vi "autosize_columns_for_text.vi"(7 "font":T1, 11 "array_to_autosize":string[][](array[string])) -> (3 "column_widths":i16[](array[numeric]))   [LabVIEW 2019]
doc: "This VI resizes each column of the table specified by Table Ref based on the widest entry of the column. Additionally, if Resize Table? is TRUE, the VI will set the table width based on the number of populated columns."
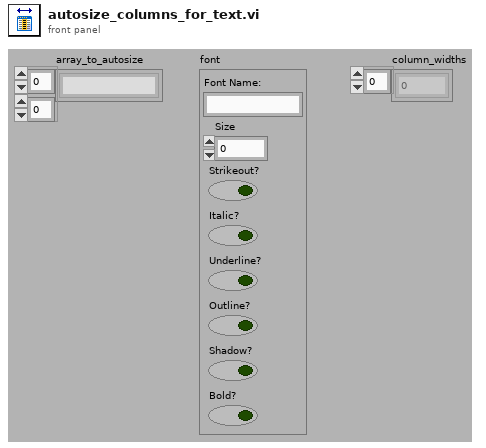
[diagram p1: front panel]
types:
  T1 = cluster{"Font Name:":string, "Size":i16, "Strikeout?":bool, "Italic?":bool, "Underline?":bool, "Outline?":bool, "Shadow?":bool, "Bold?":bool}
  T2 = enum16{"User-specified Font", "Application Font", "System Font", "Dialog Font"}
  T3 = cluster{"left":i16, "top":i16, "right":i16, "bottom":i16}
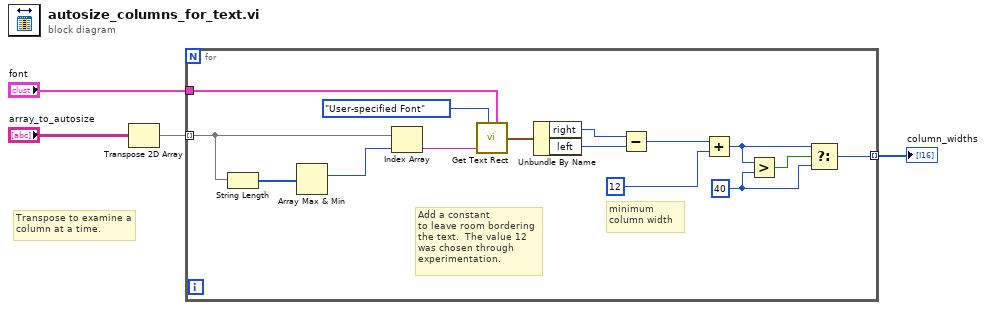
[diagram p0: block diagram]
diagram:
  # "Transpose to examine a column at a time."
  n1 = Transpose 2D Array(2D array="array_to_autosize") -> (transposed array=w4:string[][])
  n2 = for {
    tunnel: w4 -> [w19] mode=indexing
    tunnel: [w6] -> w3 mode=indexing
    tunnel: "font" -> [w5]
    w8 = i16 40 ("y")
    # "minimum\ncolumn width"
    # "Add a constant\nto leave room bordering the text.  The value 12 was chosen through experimentation."
    n3 = String Length(string=w19) -> (length=w18:i32[])
    n4 = Array Max & Min(array=w18) -> (max index (indices)=w11:i32)  [unwired: 3 out]
    n5 = Index Array(array=w19, index=w11) -> (element=w10:string)
    n6 = call <vilib>:"Get Text Rect.vi"("desired font(Application)"=T2."User-specified Font", "text"=w10, "[user-specified font]"=w5) -> ("rect"=w13:T3)  [unwired: 6 in]
    n7 = Unbundle By Name(w13) -> ("right"=w14:i16, "left"=w15:i16)
    n8 = Subtract(x=w14, y=w15) -> (x-y=w16:i16)
    n9 = Add(x=w16, y=i16 12) -> (x+y=w7:i16)
    n10 = Greater?(x=w7, y=w8) -> (0:w9:bool)
    n11 = Select(t=w7, s=w9, f=w8) -> (s? t:f=w6:i16)
  }
  "column_widths" <- w3
